vi "SequenceDiagramGraph_Create.vi"(0 "reference":refnum<class "SequenceDiagramGraph.lvclass">, 5 "error in (no error)":errorcluster, 6 "GoopReferenceIn":T1) -> (14 "reference out":refnum<class "SequenceDiagramGraph.lvclass">, 16 "# of objects":i32, 19 "error out":errorcluster)   [LabVIEW 2012, in "SequenceDiagramGraph.lvclass"]
doc: "Creates and initializes a new SequenceDiagramGraph object.\n\nThis object should be destroyed using a SequenceDiagramGraph destructor VI or a virtual base class destructor VI.\n\n[GOOP 2.3]"
uses:
  <resource>/Framework/Providers/Open_GDS/UML/SequenceDiagramGraph_class/SequenceDiagramGraph.lvclass
  <resource>/Framework/Providers/Open_GDS/UML/Graph_class/ObjectReference.ctl
  <resource>/Framework/Providers/Open_GDS/UML/ArrowHead_class/ArrowHeadType.ctl
  <resource>/Framework/Providers/Open_GDS/UML/UMLEditor/UMLEditor toolsType.ctl
  <resource>/Framework/Providers/Open_GDS/UML/CallEdge_class/CallEdge.lvclass
  <resource>/Framework/Providers/Open_GDS/UML/Graph_class/Graph.lvclass
  <resource>/Framework/Providers/Open_GDS/UML/ImplicitParameterNode_class/ImplicitParameterNode.lvclass
  <resource>/Framework/Providers/Open_GDS/UML/CallNode_class/CallNode.lvclass
  <resource>/Framework/Providers/Open_GDS/UML/NoteNode_class/NoteNode.lvclass
  <resource>/Framework/Providers/Open_GDS/UML/NoteEdge_class/NoteEdge.lvclass
  <resource>/Framework/Providers/Open_GDS/UML/ArrowHead_class/ArrowHead.lvclass
panel:
  # "The input reference should only\nbe wired when this method is called\nby a sub class constructor."
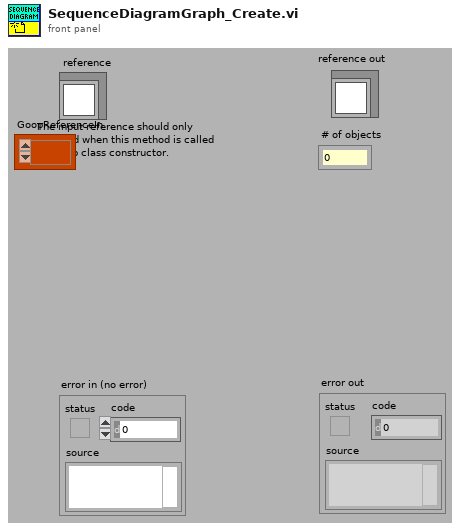
[diagram p1: front panel]
types:
  T1 = typedef "Graph.lvclass/ObjectReference.ctl" = refnum<k1>
  T2 = typedef "UMLEditor toolsType.ctl" = enum16{"CD_Select", "CD_Class", "CD_Interface", "CD_Package", "CD_Note", "CD_Dependency", "CD_Inheritance", "CD_InterfaceImp", "CD_Association", "CD_Aggregation", "CD_Composite", "CD_NoteConn", "SQD_Select", "SQD_Object", "SQD_ActionBar", "SQD_Note", "SQD_Call", "SQD_NoteConn", "UD_Select", "UD_System", "UD_Actor", "UD_UseCase", "UD_Note", "UD_Assoiciation", "UD_Generalization", "UD_GeneralizationIncludes", "UD_GeneralizationExtends", "UD_Realization", "UD_Relationship", "UD_NoteEdge", "STD_Select", "STD_State", "STD_InitailState", "STD_FinalState", "STD_StateTransation", "STD_Note", "STD_NoteEdge"}
  T3 = typedef "ArrowHead.lvclass/ArrowHeadType.ctl" = enum16{"NONE", "TRIANGLE", "BLACK_TRIANGLE", "V", "HALF_V", "DIAMOND", "BLACK_DIAMOND"}
  T4 = typedef "SequenceDiagramGraph.lvclass/ClassAttributes.ctl" = cluster{"Base class":T5}
  T5 = typedef "Graph.lvclass/ClassAttributes.ctl" = cluster{"NODE_PROT":refnum<class "AbstractNode.lvclass">[], "NodeNames":string[], "EDGE_PROT":refnum<class "AbstractEdge.lvclass">[], "EdgeNames":string[]}
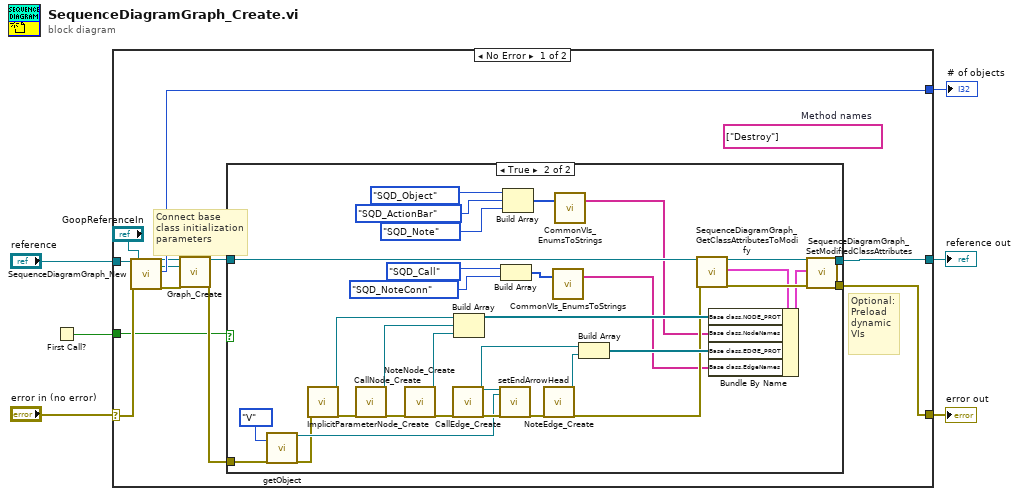
[diagram p0: block diagram]
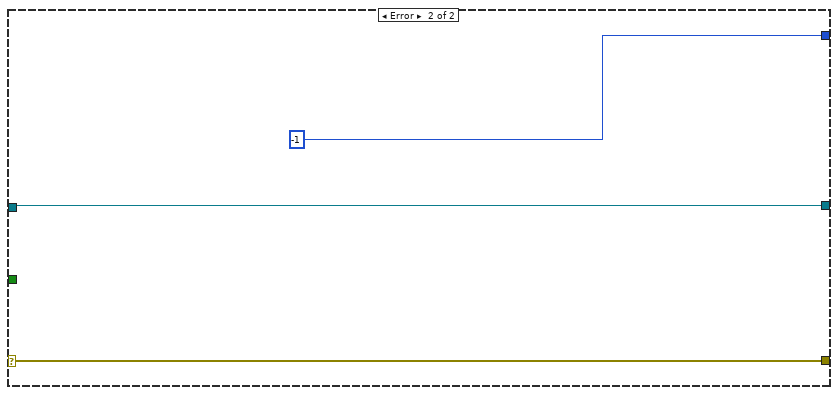
[diagram p3: hidden frame]
diagram:
  n1 = First Call?() -> (First Call?: T/F=w1:bool)
  n2 = case shown="No Error" "error in (no error)" {
    selector: "error in (no error)" -> [w18 w55]
    tunnel: [w13 w54] -> w6
    tunnel: [w12 w55] -> w5
    tunnel: [w17 -1 ("Nr of open handles")] -> w4
    tunnel: "reference" -> [w16 w54]
    tunnel: w1 -> [w9 _]
    frame No Error {
      (unwired) string[] ["Destroy"]  # Method names
      # "Optional:\nPreload\ndynamic\nVIs"
      # "Connect base\nclass initialization\nparameters"
      n3 = call <resource>:"SequenceDiagramGraph_New.vi"("reference in"=w16, "error in (no error)"=w18, "GoopReferenceIn"="GoopReferenceIn") -> ("GoopReferenceOut"=w7:T1, "reference out"=w15:refnum<class "SequenceDiagramGraph.lvclass">, "# of objects"=w17:i32, "error out"=w11:errorcluster)  [unwired: 2 in, 11 out]
      n4 = call <resource>:"Graph_Create.vi"("reference"=w15, "error in (no error)"=w11, "GoopReferenceIn"=w7) -> ("reference out"=w14:refnum<class "SequenceDiagramGraph.lvclass">, "error out"=w10:errorcluster)  [unwired: 15 out]
      n5 = case shown="True" w9 {
        tunnel: w14 -> [w20 w52]
        tunnel: [w19 w48] -> w12
        tunnel: [w20 w47] -> w13
        tunnel: w10 -> [w19 w31]
        frame False {
        }
        frame True {
          n6 = call <resource>:"getObject.vi"("arrowHead"=ArrowHeadType."V", "error in (no error)"=w31) -> ("reference out"=w33:refnum<class "ArrowHead.lvclass">, "error out"=w30:errorcluster)  [unwired: 16 out]
          n7 = call <resource>:"ImplicitParameterNode_Create.vi"("error in (no error)"=w30) -> ("reference out"=w44:refnum<class "ImplicitParameterNode.lvclass">, "error out"=w45:errorcluster)  [unwired: 2 in, 15 out]
          n8 = call <resource>:"CallNode_Create.vi"("error in (no error)"=w45) -> ("reference out"=w43:refnum<class "CallNode.lvclass">, "error out"=w46:errorcluster)  [unwired: 2 in, 15 out]
          n9 = call <resource>:"NoteNode_Create.vi"("error in (no error)"=w46) -> ("reference out"=w42:refnum<class "NoteNode.lvclass">, "error out"=w40:errorcluster)  [unwired: 2 in, 15 out]
          n10 = call <resource>:"CallEdge_Create.vi"("error in (no error)"=w40) -> ("reference out"=w36:refnum<class "CallEdge.lvclass">, "error out"=w35:errorcluster)  [unwired: 1 in, 16 out]
          n11 = Build Array(w44, w43, w42) -> (w41:refnum<class "RectangularNode.lvclass">[])
          n12 = call-dynamic "setEndArrowHead.vi"("reference"=w36, "endArrowHead"=w33, "error in (no error)"=w35) -> ("error out"=w34:errorcluster)  [unwired: 15 in, 1 out]
          n13 = Build Array(UMLEditor_toolsType."SQD_Call" ("tool"), UMLEditor_toolsType."SQD_NoteConn" ("tool")) -> (w22:T2[])
          n14 = Build Array(UMLEditor_toolsType."SQD_Object" ("tool"), UMLEditor_toolsType."SQD_ActionBar" ("tool"), UMLEditor_toolsType."SQD_Note" ("tool")) -> (w29:T2[])
          n15 = call <resource>:"NoteEdge_Create.vi"("error in (no error)"=w34) -> ("reference out"=w39:refnum<class "NoteEdge.lvclass">, "error out"=w37:errorcluster)  [unwired: 1 in, 16 out]
          n16 = call <resource>:"CommonVIs_EnumsToStrings.vi"("ArrayEnumVariantIn"=w22) -> ("EnumItems(string)"=w21:string[])  [unwired: 2 in, 16 out]
          n17 = call <resource>:"CommonVIs_EnumsToStrings.vi"("ArrayEnumVariantIn"=w29) -> ("EnumItems(string)"=w26:string[])  [unwired: 2 in, 16 out]
          n18 = Build Array(w36, w39) -> (w38:refnum<class "GeneralPathEdge.lvclass">[])
          n19 = call <resource>:"SequenceDiagramGraph_GetClassAttributesToModify.vi"("reference in"=w52, "error in (no error)"=w37) -> ("reference out"=w51:refnum<class "SequenceDiagramGraph.lvclass">, "Class attributes"=w50:T4, "error out"=w53:errorcluster)  [unwired: 1 in, 14 out]
          n20 = Bundle By Name(cluster=w50, "Base class.NODE_PROT"=w41, "Base class.NodeNames"=w26, "Base class.EDGE_PROT"=w38, "Base class.EdgeNames"=w21) -> (w49:T4)
          n21 = call <resource>:"SequenceDiagramGraph_SetModifiedClassAttributes.vi"("reference in"=w51, "Class attributes"=w49, "error in (no error)"=w53) -> ("reference out"=w47:refnum<class "SequenceDiagramGraph.lvclass">, "error out"=w48:errorcluster)  [unwired: 2 in, 13 out]
        }
      }
    }
    frame Error {
    }
  }
  "error out" <- w5
  "reference out" <- w6
  "# of objects" <- w4
